vi "ClearMotionError.vi"(5 "error in (no error)":errorcluster) -> (19 "error out":errorcluster)   [LabVIEW 2020]
doc: "Clears Motion Error from controller (Error 10)"
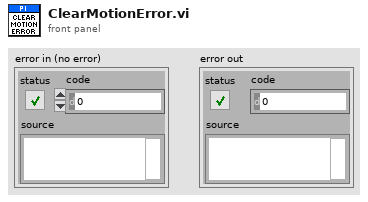
[diagram p1: front panel]
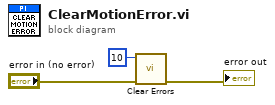
[diagram p0: block diagram]
diagram:
  n1 = call "Clear Errors.vi"("error in (no error)"="error in (no error)", "specific error code to clear (0: all)"=10) -> ("error out"=→"error out":errorcluster)  [unwired: 5 out]
